vi "FGV Hangup.vi"(6 "Aktion":T4, 7 "Protokoll":T1 {"Messgasdruck Amium" format="%.2f"; "FID Mittelwert E" format="%.2f"; "FID Mittelwert 0" format="%.2f"}, 8 "error in (no error)":errorcluster caption="Fehler (Eingang, kein Fehler)", 9 "Textname:":string, 10 "Pfad:":path=path "D:/IAG_Data/Log", 11 "Hangup Settings":T2 {"Grenzwert: C1" format="%#.1f"; "Spankonzentration [ppm]" format="%#.1f"; "Messbereich" items=["---", "0-500", "0-5000", "0-10000"]; "Grenze" items=["Manuell", "Auto"]; "Grenzwert:" format="%#.1f"; "Grenzwert manuell:" format="%#.1f"; "Datenerfassungszeit:" format="%#.1f"; "Nullgas Aufschaltzeit:" format="%#.1f"; "Spangas Aufschaltzeit:" format="%#.1f"; "Aufschaltpunkt" items=["Filterblock", "Analyzer directly", "PNS"]; "Kalibriergas" items=["Stickstoff", "CO", "C3H8", "CH4", "O2", "", "", "", "", "", "", "", ""]}) -> (0 "error out":errorcluster caption="Fehler (Ausgang)", 1 "Textname:":string, 2 "Pfad:":path, 3 "Hangup Settings":T2 {"Grenzwert: C1" format="%#.1f"; "Spankonzentration [ppm]" format="%#.1f"; "Messbereich" items=["---", "0-500", "0-5000", "0-10000"]; "Grenze" items=["Manuell", "Auto"]; "Grenzwert:" format="%#.1f"; "Grenzwert manuell:" format="%#.1f"; "Datenerfassungszeit:" format="%#.1f"; "Nullgas Aufschaltzeit:" format="%#.1f"; "Spangas Aufschaltzeit:" format="%#.1f"; "Aufschaltpunkt" items=["Filterblock", "Analyzer directly", "PNS"]; "Kalibriergas" items=["Stickstoff", "CO", "C3H8", "CH4", "O2", "", "", "", "", "", "", "", ""]}, 5 "Protokoll":T1 {"Messgasdruck Amium" format="%.2f"; "FID Mittelwert E" format="%.2f"; "FID Mittelwert 0" format="%.2f"})   [LabVIEW 2020, in "Hangup Check.lvlib"]
uses:
  Hangup Check.lvlib
  AktionFGV Hangup.ctl
  HangupSettings.ctl
  Visualisierungs Elemente/Auswahlfeld.ctl
  Protokoll.ctl
  Allgemein/allgemeine Sub-VIs.lvlib
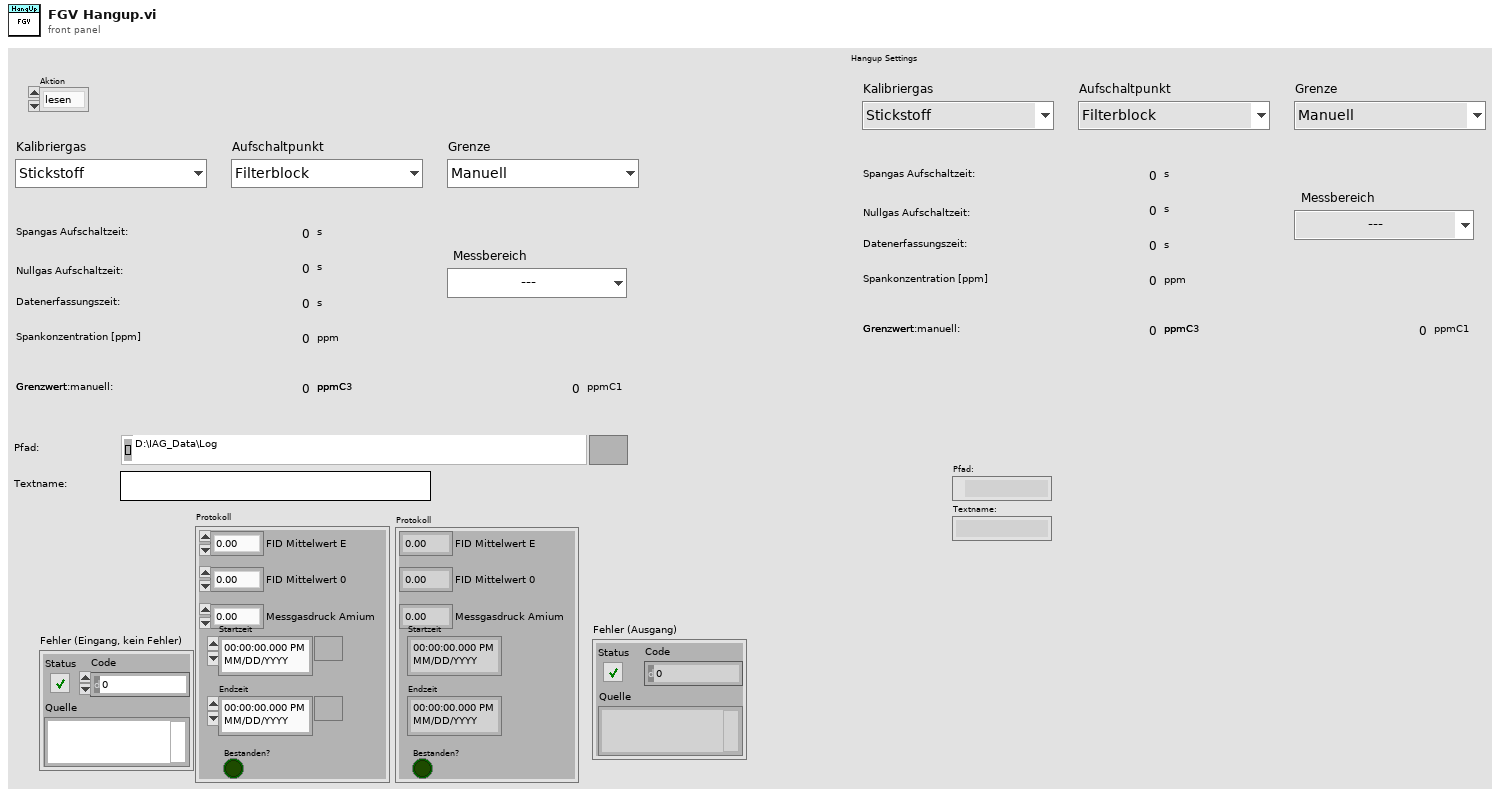
[diagram p1: front panel]
types:
  T1 = typedef "Hangup Check.lvlib/Protokoll.ctl" = cluster{"FID Mittelwert 0":sgl, "FID Mittelwert E":sgl, "Messgasdruck Amium":sgl, "Startzeit":timestamp, "Endzeit":timestamp, "Bestanden?":bool}
  T2 = typedef "Hangup Check.lvlib/HangupSettings.ctl" = cluster{"Kalibriergas":T3, "Aufschaltpunkt":T3, "Spangas Aufschaltzeit:":sgl, "Nullgas Aufschaltzeit:":sgl, "Datenerfassungszeit:":sgl, "Grenzwert manuell:":sgl, "Grenzwert:":sgl, "Grenze":T3, "Messbereich":T3, "Spankonzentration [ppm]":sgl, "Grenzwert: C1":sgl}
  T3 = typedef "Auswahlfeld.ctl" = u16
  T4 = typedef "Hangup Check.lvlib/AktionFGV Hangup.ctl" = enum16{"lesen", "Hangup Settings", "Protokoll", "Pfad", "laden", "speichern"}
  T5 = cluster{"Hangup Settings":T2, "Pfad:":path, "Textname:":string}
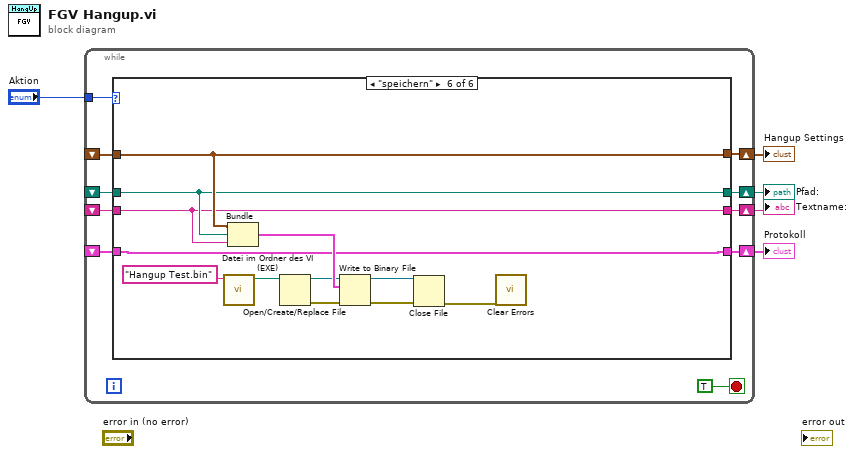
[diagram p0: block diagram]
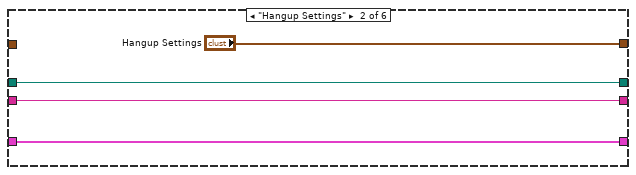
[diagram p3: hidden frame]
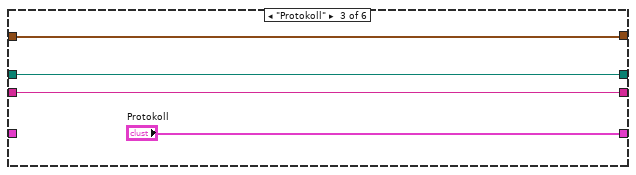
[diagram p4: hidden frame]
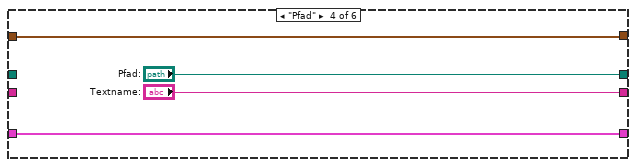
[diagram p5: hidden frame]
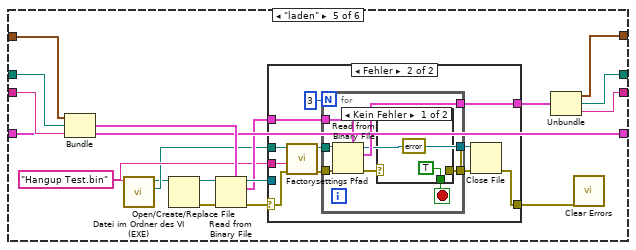
[diagram p6: hidden frame]
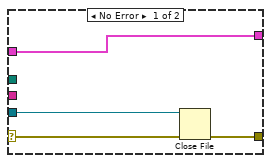
[diagram p7: hidden frame]
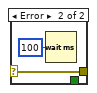
[diagram p8: hidden frame]
diagram:
  n1 = while {
    tunnel: "Aktion" -> [w15]
    shift-right: [w14] -> w4
    shift-left: _ -> [w13]
    shift-right: [w12] -> w3
    shift-left: _ -> [w10]
    shift-right: [w11] -> w2
    shift-left: _ -> [w9]
    shift-right: [w7] -> w1
    shift-left: _ -> [w6]
    stop <- TRUE stop-if-true
    n2 = case shown="\"speichern\"" w15 {
      tunnel: [w19 "Hangup Settings" w27 w31 w45 w87] -> w14
      tunnel: w13 -> [w19 _ w27 w31 w49 w87]
      tunnel: [w18 w22 w26 "Pfad:" w44 w86] -> w12
      tunnel: [w17 w21 w25 "Textname:" w43 w85] -> w11
      tunnel: w10 -> [w18 w22 w26 _ w48 w86]
      tunnel: w9 -> [w17 w21 w25 _ w47 w85]
      tunnel: [w16 w20 "Protokoll" w28 w42 w83] -> w7
      tunnel: w6 -> [w16 w20 _ w28 w42 w83]
      frame "lesen", Default {
      }
      frame "Hangup Settings" {
      }
      frame "Protokoll" {
      }
      frame "Pfad" {
      }
      frame "laden" {
        w36 = "Hangup Test.bin" ("Dateiname")
        n3 = Bundle("Hangup Settings"=w49, "Pfad:"=w48, "Textname:"=w47) -> (w46:T5)  [unwired: 1 in]
        n4 = call "Datei im Ordner des VI (EXE).vi"("Dateiname"=w36) -> ("Ordner des Haupt-VIs"=w35:path, "Dateipfad im Ordner des Haupt-VIs"=w34:path)  [unwired: 8 in, 1 out]
        n5 = Open/Create/Replace File(file path (use dialog)=w34) -> (refnum out=w33:refnum<file>, error out=w32:errorcluster)  [unwired: 5 in, 1 out]
        n6 = Read from Binary File(5:w46, 8:w32, 11:w33) -> (0:w41:errorcluster, 2:w39:T5, 3:w40:refnum<file>)  [unwired: 3 in, 1 out]
        n7 = case shown="Fehler" w41 {
          selector: w41 -> [w52 w56]
          tunnel: w35 -> [_ w57]
          tunnel: w39 -> [w53 w55]
          tunnel: [w53 w63] -> w38
          tunnel: [w50 w61] -> w37
          tunnel: w40 -> [w51 _]
          tunnel: w36 -> [_ w54]
          frame No Error {
            n8 = Close File(refnum=w51, error in=w52) -> (error out=w50:errorcluster)  [unwired: 1 out]
          }
          frame Error {
            n9 = call "Factorysettings Pfad.vi"("error in (no error)"=w56, "Dateiname"=w54, "Ordner des Haupt-VIs"=w57) -> ("error out"=w58:errorcluster, "Pfad Factorysettings"=w59:path)  [unwired: 7 in]
            n10 = for {
              N: 3 -> [_]
              tunnel: w58 -> [w70]
              tunnel: w59 -> [w69]
              tunnel: [w68] -> w63
              tunnel: [w67] -> w62
              tunnel: [w66] -> w60
              tunnel: w55 -> [w65]
              stop <- w71 stop-if-true
              n11 = Read from Binary File(5:w65, 8:w70, 11:w69) -> (0:w72:errorcluster, 2:w68:T5, 3:w66:refnum<file>)  [unwired: 3 in, 1 out]
              n12 = case shown="Kein Fehler" w72 {
                selector: w72 -> [_ w75]
                tunnel: [TRUE _] -> w71
                tunnel: [errorcluster {"status"=FALSE, "code"=0, "source"=""} ("error IO") w75] -> w67
                frame No Error {
                }
                frame Error {
                  n13 = Wait (ms)(milliseconds to wait=u32 100 ("Zu wartende ms")) -> ()  [unwired: 1 out]
                }
              }
            }
            n14 = Close File(refnum=w60, error in=w62) -> (error out=w61:errorcluster)  [unwired: 1 out]
          }
        }
        n15 = Unbundle(w38) -> ("Hangup Settings"=w45:T2, "Pfad:"=w44:path, "Textname:"=w43:string)
        n16 = call <vilib>:"Clear Errors.vi"("error in (no error)"=w37) -> ()  [unwired: 5 in, 2 out]
      }
      frame "speichern" {
        n17 = call "Datei im Ordner des VI (EXE).vi"("Dateiname"="Hangup Test.bin") -> ("Dateipfad im Ordner des Haupt-VIs"=w82:path)  [unwired: 8 in, 2 out]
        n18 = Bundle("Hangup Settings"=w87, "Pfad:"=w86, "Textname:"=w85) -> (w84:T5)  [unwired: 1 in]
        n19 = Open/Create/Replace File(file path (use dialog)=w82) -> (refnum out=w81:refnum<file>, error out=w80:errorcluster)  [unwired: 5 in, 1 out]
        n20 = Write to Binary File(file (use dialog)=w81, data=w84, error in=w80) -> (refnum out=w78:refnum<file>, error out=w79:errorcluster)  [unwired: 3 in, 1 out]
        n21 = Close File(refnum=w78, error in=w79) -> (error out=w77:errorcluster)  [unwired: 1 out]
        n22 = call <vilib>:"Clear Errors.vi"("error in (no error)"=w77) -> ()  [unwired: 5 in, 2 out]
      }
    }
  }
  "Hangup Settings" <- w4
  "Pfad:" <- w3
  "Textname:" <- w2
  "Protokoll" <- w1
